vi "Manual_DAC_ramp.vi"() -> ()   [LabVIEW 2013]
uses:
  <vilib>/rvi/interface/nirviCloseFPGA/nirviCloseFPGA.xnode
  FPGA Bitfiles/fpga-clean.lvproj_FPGA Target 2_lock-in(FPGA).vi.lvbit
  fpga-bitfile-ref.ctl
  <vilib>/FPGAPlugInAG/sbRIO-9612/niLvFpga_Close_sbRIO-9612.vi
panel:
  in  "min":dbl=-2.0
  in  "max":dbl=0.3
  in  "Set mode":bool
  in  "DAC control":dbl[][](array[numeric])=[[0.0, 0.0, 0.0, 0.0, 0.0, 0.0, 0.0, 0.0], [0.0, 0.0, 0.0, 0.0, 0.0, 0.0, 0.0, 0.0], [0.0, 0.0, 0.0, 0.0, 0.0, 0.0, 0.0, 0.0], [0.0, 0.0, 0.0, 0.0, 0.0, 0.0, 0.0, 0.0], [0.0, 0.0, 0.0, 0.0, 0.0, 0.0, 0.0, 0.0], [0.0, 0.0, 0.0, 0.0, 0.0, 0.0, 0.0, 0.0], [0.0, 0.0, 0.0, 0.0, 0.0, 0.0, 0.0, 0.0], [0.0, 0.0, 0.0, 0.0, 0.0, 0.0, 0.0, 0.0]]
  in  "IP Adress FPGA":string="192.168.0.3"
  in  "Delay(ms)":u8=1
  in  "Busses to be used":bool[](array[boolean])=[TRUE, FALSE, TRUE, FALSE, TRUE, FALSE, FALSE, FALSE]
  # "Read"
  # "Set"
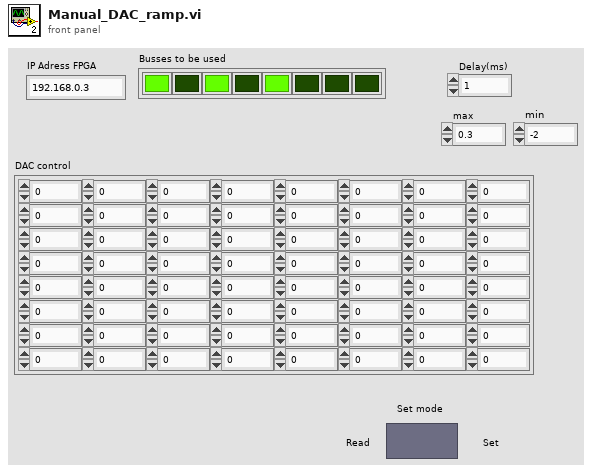
[diagram p1: front panel]
types:
  T1 = enum16{"frequency", "channel", "amplitude", "inhibate"}
  T2 = enum8{"start movement", "buses to use", "delay", "value", "stop", ""}
  T3 = typedef "fpga-bitfile-ref.ctl" = refnum<k20>
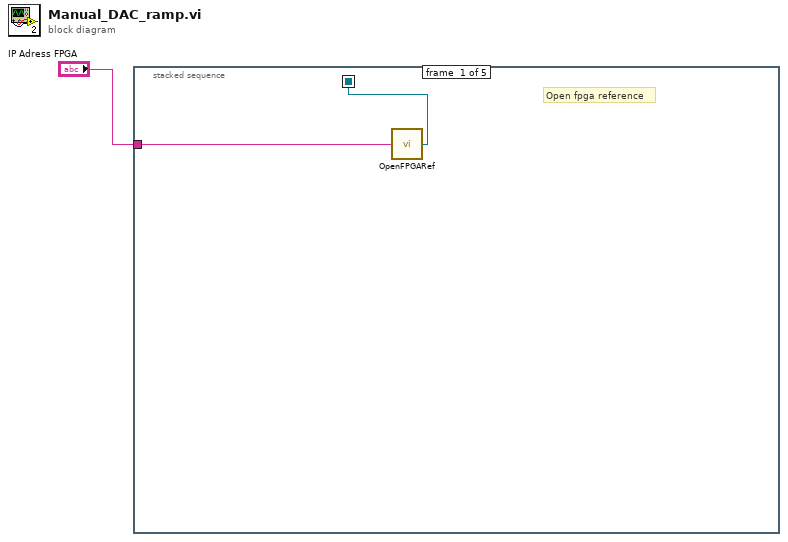
[diagram p0: block diagram]
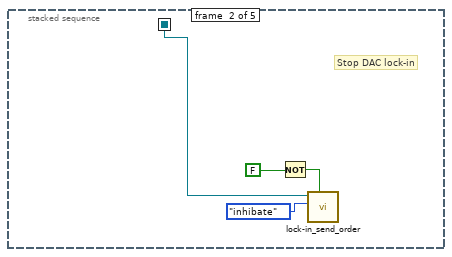
[diagram p2: hidden frame]
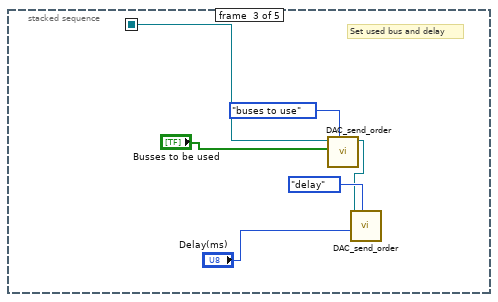
[diagram p3: hidden frame]
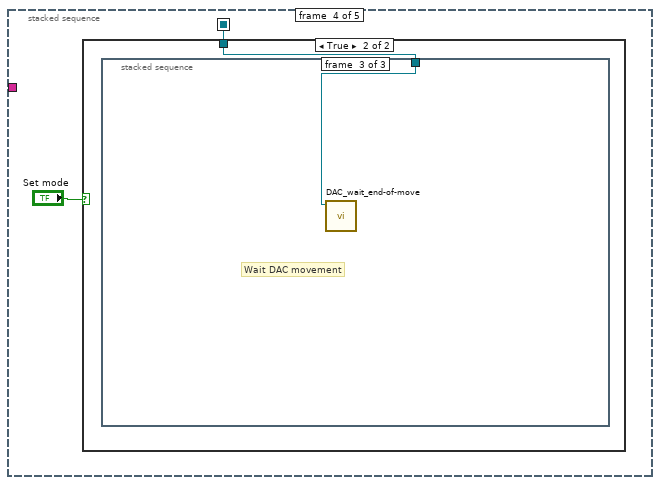
[diagram p4: hidden frame]
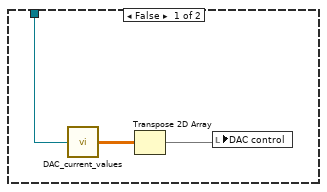
[diagram p5: hidden frame]
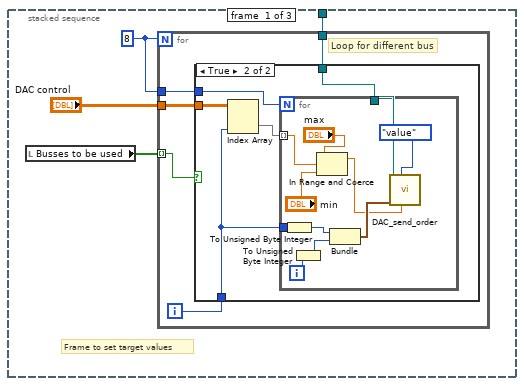
[diagram p6: hidden frame]
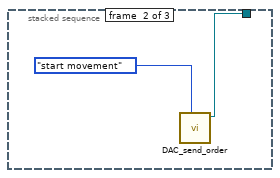
[diagram p8: hidden frame]
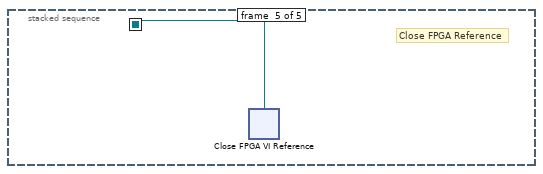
[diagram p9: hidden frame]
diagram:
  n1 = stacked-sequence {
    seq-local: [w2 _ _ _ _] -> [_ w4 w11 w14 w48]
    tunnel: "IP Adress FPGA" -> [w3 _ _ _ _]
    frame #0 {
      # "Open fpga reference"
      n2 = call "OpenFPGARef.vi"("IP Address"=w3) -> ("FPGA VI Reference Out"=w2:T3)
    }
    frame #1 {
      # "Stop DAC lock-in"
      n3 = Not(x=FALSE) -> (.not. x?=w6:bool)
      n4 = call "lock-in_send_order.vi"("inhibate?"=w6, "order"=T1."inhibate", "FPGA VI Reference In"=w4) -> ()  [unwired: 4 in, 5 out]
    }
    frame #2 {
      # "Set used bus and delay"
      n5 = call "DAC_send_order.vi"("order"=T2."buses to use", "buses to use"="Busses to be used", "FPGA VI Reference In"=w11) -> ("FPGA VI Reference Out"=w8:T3)  [unwired: 8 in]
      n6 = call "DAC_send_order.vi"("order"=T2."delay", "delay between steps (ms)"="Delay(ms)", "FPGA VI Reference In"=w8) -> ()  [unwired: 8 in, 1 out]
    }
    frame #3 {
      n7 = case shown="True" "Set mode" {
        tunnel: w14 -> [w18 w19]
        frame False {
          n8 = call "DAC_current_values.vi"("FPGA Ref"=w18) -> ("DAC values"=w17:sgl[][])
          n9 = Transpose 2D Array(2D array=w17) -> (transposed array=w16:sgl[][])
          n10 = local write "DAC control"(w16) -> ()
        }
        frame True {
          n11 = stacked-sequence {
            tunnel: w19 -> [w20 w45 w47]
            frame #0 {
              w21 = 8
              # "Frame to set target values"
              n12 = local read "Busses to be used"() -> (w23:bool[])
              n13 = for {
                N: w21 -> [_]
                tunnel: w23 -> [w28] mode=indexing
                tunnel: "DAC control" -> [w27]
                tunnel: w21 -> [w25]
                tunnel: w20 -> [w24]
                i -> [w26]
                # "Loop for different bus"
                n14 = case shown="True" w28 {
                  tunnel: w27 -> [_ w33]
                  tunnel: w26 -> [_ w30]
                  tunnel: w25 -> [_ w31]
                  tunnel: w24 -> [_ w29]
                  frame False {
                  }
                  frame True {
                    n15 = Index Array(array=w33, index (col)=w30) -> (element=w32:dbl[])  [unwired: 1 in]
                    n16 = for {
                      N: w31 -> [_]
                      tunnel: w32 -> [w37] mode=indexing
                      tunnel: w30 -> [w44]
                      tunnel: w29 -> [w39]
                      i -> [w43]
                      n17 = To Unsigned Byte Integer(number=w44) -> (unsigned 8bit integer=w41:u8)
                      n18 = To Unsigned Byte Integer(number=w43) -> (unsigned 8bit integer=w42:u8)
                      n19 = In Range and Coerce(upper limit="max", x=w37, lower limit="min") -> (coerced(x)=w36:dbl)  [unwired: 1 out]
                      n20 = Bundle(w41, w42) -> (w38:cluster{u8, u8})  [unwired: 1 in]
                      n21 = call "DAC_send_order.vi"("DAC goto value"=w36, "order"=T2."value", "Cluster"=w38, "FPGA VI Reference In"=w39) -> ()  [unwired: 7 in, 1 out]
                    }
                  }
                }
              }
            }
            frame #1 {
              n22 = call "DAC_send_order.vi"("order"=T2."start movement", "FPGA VI Reference In"=w45) -> ()  [unwired: 9 in, 1 out]
            }
            frame #2 {
              # "Wait DAC movement"
              n23 = call "DAC_wait_end-of-move.vi"("FPGA VI Reference In"=w47) -> ()  [unwired: 11 out]
            }
          }
        }
      }
    }
    frame #4 {
      # "Close FPGA Reference"
      n24 = xnode "Close FPGA VI Reference"("FPGA VI Reference In"=w48) -> ()  [unwired: 1 in, 1 out]
    }
  }
